vi "Go.vi"(9 "Timing Data":dbl[](array[numeric]), 10 "Control In":T1, 11 "C4 Dispense in":refnum<class "Iterative Dispense.lvclass">) -> (2 "Control Out":T1, 3 "C4 Dispense Out":refnum<class "Iterative Dispense.lvclass">)   [LabVIEW 2020, in "Iterative Dispense.lvclass"]
uses:
  Iterative Dispense.lvclass
  Controller/Controllers.ctl
  Controller/I-O/I-O.lvclass
  Controller/Dispenser/Dispenser.lvclass
  C:/Program Files (x86)/Aerotech/A3200/LabVIEW/2010/Bin/Aerotech.A3200.dll
  Program Files (x86)/Aerotech/A3200/LabVIEW/2010/Bin/Aerotech.A3200.dll
  Iterative Dispense.lvclass/Iterative Dispense.ctl
  Controller/Motion/A3200/A3200.lvclass
  Controller/Controller.lvclass
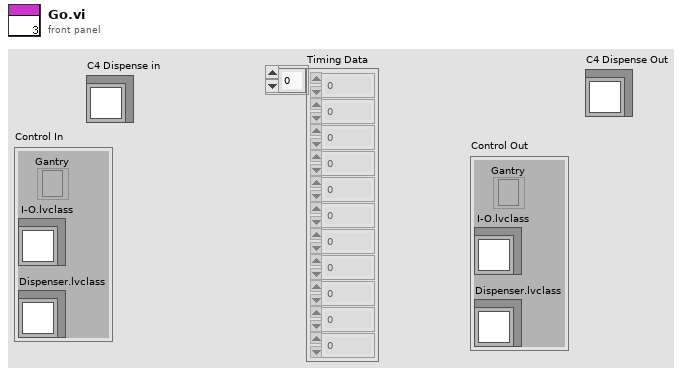
[diagram p1: front panel]
types:
  T1 = typedef "Controller.lvclass/Controllers.ctl" = cluster{"I-O.lvclass":refnum<class "I-O.lvclass">, "Dispenser.lvclass":refnum<class "Dispenser.lvclass">, "Gantry":refnum<k24>}
  T2 = typedef "Iterative Dispense.lvclass/Glue Step Enum.ctl" = enum16{"Baseplate to Kapton", "Kapton to Sensor"}
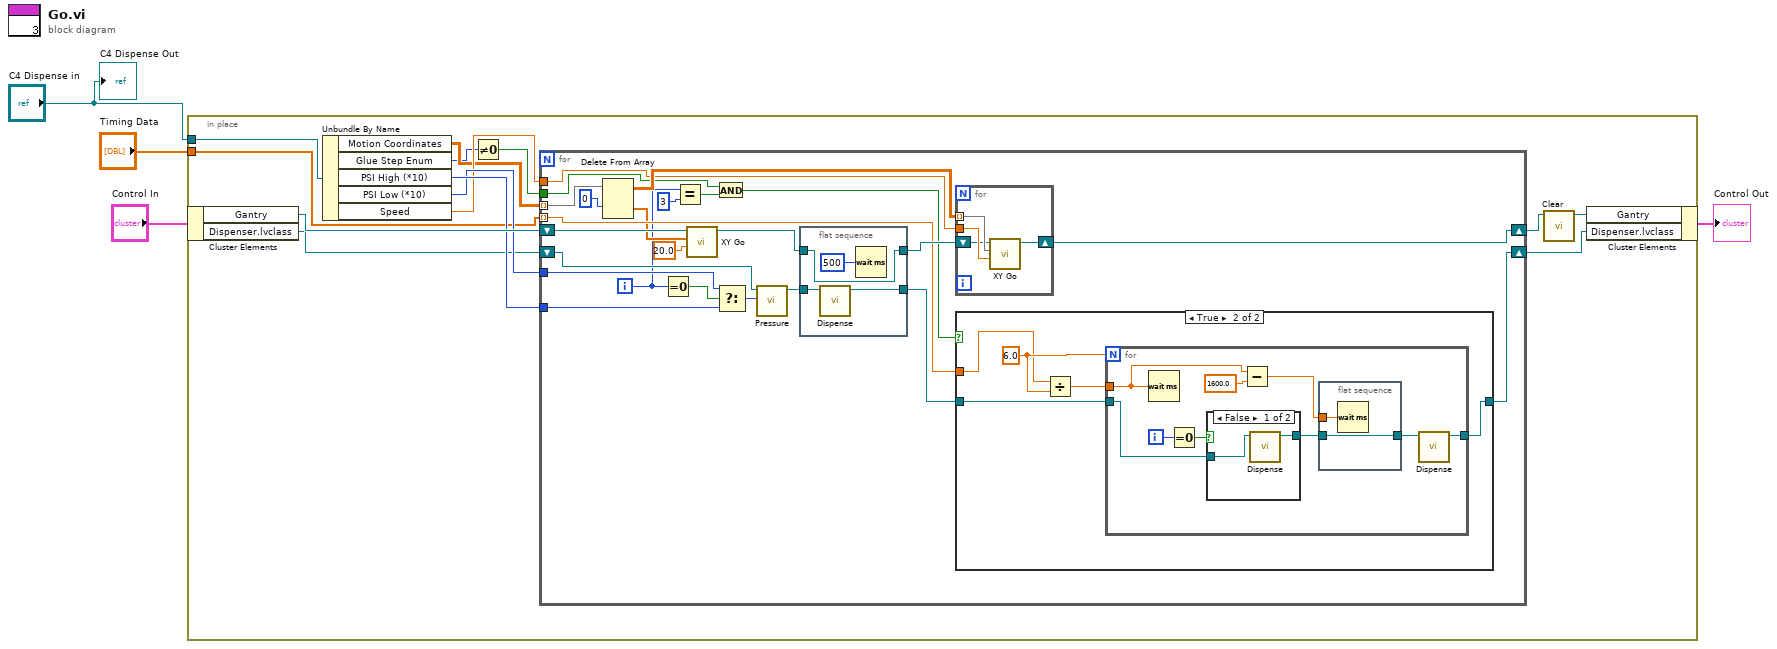
[diagram p0: block diagram]
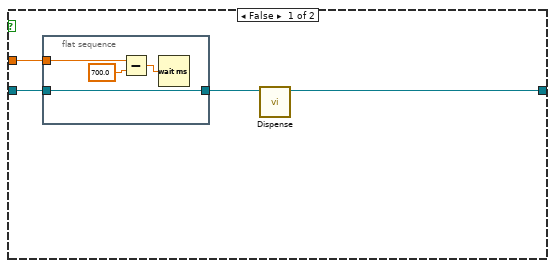
[diagram p2: hidden frame]
diagram:
  n1 = in-place {
    in-place-border: "C4 Dispense in" -> [w14]
    in-place-border: "Timing Data" -> [w10]
    n2 = in-place-cluster #1("Control In") -> ("Gantry"=w16:refnum<k24>, "Dispenser.lvclass"=w7:refnum<class "Dispenser.lvclass">)
    n3 = Unbundle By Name(w14) -> ("Motion Coordinates"=w9:dbl[][][], "Glue Step Enum"=w6:T2, "PSI High (*10)"=w13:i32, "PSI Low (*10)"=w12:i32, "Speed"=w11:dbl)
    n4 = Not Equal To 0?(x=w6) -> (x != 0?=w17:bool)
    n5 = for {
      tunnel: w9 -> [w37] mode=indexing
      tunnel: w17 -> [w31]
      tunnel: w11 -> [w29]
      tunnel: w10 -> [w28] mode=indexing
      tunnel: w12 -> [w27]
      tunnel: w13 -> [w26]
      shift-right: [w41] -> w8
      shift-left: w16 -> [w25]
      shift-right: [w38] -> w15
      shift-left: w7 -> [w19]
      i -> [w18]
      # "Executes C4 Symmetric Motion"
      n6 = Delete From Array(array=w37, index (row)=0) -> (deleted portion=w23:dbl[], array with subset deleted=w35:dbl[][])  [unwired: 2 in]
      n7 = Equal To 0?(x=w18) -> (x = 0?=w30:bool)
      n8 = Equal?(x=w18, y=3) -> (x = y?=w39:bool)
      n9 = call "XY Go.vi"("Speed"=20.0 ("speed"), "XY"=w23, "Gantry In"=w25) -> ("Gantry Out"=w24:refnum<k24>)  [unwired: 7 in, 1 out]
      n10 = And(x=w31, y=w39) -> (x .and. y?=w32:bool)
      n11 = Select(t=w27, s=w30, f=w26) -> (s? t:f=w20:i32)
      n12 = call-dynamic "Pressure.vi"("Pressure"=w20, "Dispenser in"=w19) -> ("Dispenser out"=w21:refnum<class "Dispenser.lvclass">)  [unwired: 8 in, 1 out]
      n13 = flat-sequence {
        tunnel: w21 -> [w70]
        tunnel: w24 -> [w71]
        tunnel: [w71] -> w34
        tunnel: [w69] -> w33
        frame #0 {
          n14 = call-dynamic "Dispense.vi"("Dispenser in"=w70) -> ("Dispenser out"=w69:refnum<class "Dispenser.lvclass">)  [unwired: 9 in, 1 out]
          n15 = Wait (ms)(milliseconds to wait=u32 500) -> ()  [unwired: 1 out]
        }
      }
      n16 = for {
        tunnel: w29 -> [w75]
        tunnel: w35 -> [w76] mode=indexing
        shift-right: [w73] -> w41
        shift-left: w34 -> [w74]
        n17 = call "XY Go.vi"("Speed"=w75, "XY"=w76, "Gantry In"=w74) -> ("Gantry Out"=w73:refnum<k24>)  [unwired: 7 in, 1 out]
      }
      n18 = case shown="True" w32 {
        tunnel: w28 -> [w45 w50]
        tunnel: w33 -> [w44 w53]
        tunnel: [w42 w52] -> w38
        frame False {
          n19 = flat-sequence {
            tunnel: w44 -> [w47]
            tunnel: w45 -> [w46]
            tunnel: [w47] -> w43
            frame #0 {
              n20 = Subtract(x=w46, y=700.0) -> (x-y=w49:dbl)
              n21 = Wait (ms)(milliseconds to wait=w49) -> ()  [unwired: 1 out]
            }
          }
          n22 = call-dynamic "Dispense.vi"("Dispenser in"=w43) -> ("Dispenser out"=w42:refnum<class "Dispenser.lvclass">)  [unwired: 9 in, 1 out]
        }
        frame True {
          w51 = 6.0 ("y")
          # "Leaves Space for Silver Epoxy"
          n23 = Divide(x=w50, y=w51) -> (x/y=w54:dbl)
          n24 = for {
            N: w51 -> [_]
            tunnel: w54 -> [w61]
            tunnel: w53 -> [w60]
            tunnel: [w56] -> w52
            i -> [w58]
            n25 = Wait (ms)(milliseconds to wait=w61) -> ()  [unwired: 1 out]
            n26 = Equal To 0?(x=w58) -> (x = 0?=w57:bool)
            n27 = case shown="False" w57 {
              tunnel: w60 -> [w64 w66]
              tunnel: [w65 w66] -> w59
              frame False {
                n28 = call-dynamic "Dispense.vi"("Dispenser in"=w64) -> ("Dispenser out"=w65:refnum<class "Dispenser.lvclass">)  [unwired: 9 in, 1 out]
              }
              frame True {
              }
            }
            n29 = Subtract(x=w61, y=1600.0) -> (x-y=w62:dbl)
            n30 = flat-sequence {
              tunnel: w62 -> [w68]
              tunnel: w59 -> [w67]
              tunnel: [w67] -> w55
              frame #0 {
                n31 = Wait (ms)(milliseconds to wait=w68) -> ()  [unwired: 1 out]
              }
            }
            n32 = call-dynamic "Dispense.vi"("Dispenser in"=w55) -> ("Dispenser out"=w56:refnum<class "Dispenser.lvclass">)  [unwired: 9 in, 1 out]
          }
        }
      }
    }
    n33 = call "Clear.vi"("Gantry In"=w8) -> ("Gantry Out"=w5:refnum<k24>)  [unwired: 9 in, 1 out]
    n34 = in-place-cluster #1("Gantry"=w5, "Dispenser.lvclass"=w15) -> (→"Control Out":T1)
  }
  "C4 Dispense Out" <- "C4 Dispense in"
